vi "Read Theme Data.vi"(8 "error in (no error)":errorcluster, 11 "Appearance Actor in":refnum<class "Appearance Actor.lvclass">) -> (0 "error out":errorcluster, 2 "Theme Data":T1, 3 "Appearance Actor out":refnum<class "Appearance Actor.lvclass">)   [LabVIEW 2021, in "Appearance Actor.lvlib" / "Appearance Actor.lvclass"]
uses:
  Appearance Actor.lvclass
  Typedefs/Theme Data--cluster.ctl
  <vilib>/Utility/config.llb/Config Data RefNum.ctl
  Appearance Actor.lvclass/Appearance Actor.ctl
  <vilib>/Utility/config.llb/NI_LVConfig.lvlib
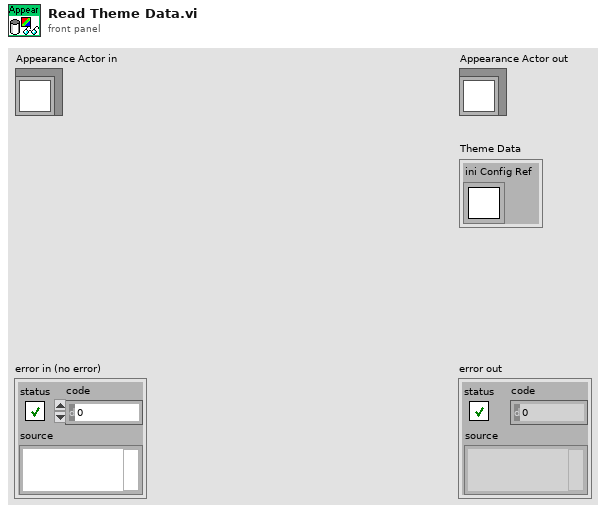
[diagram p1: front panel]
types:
  T1 = typedef "Appearance Actor.lvlib/Appearance Actor.lvclass/Theme Data--cluster.ctl" = cluster{"ini Config Ref":T2}
  T2 = typedef "NI_LVConfig.lvlib/Config Data RefNum.ctl" = refnum<k1>
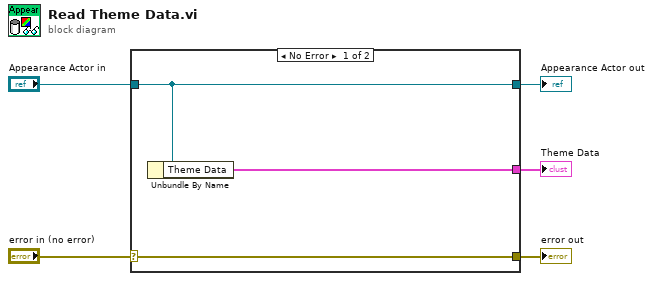
[diagram p0: block diagram]
diagram:
  n1 = case shown="No Error" "error in (no error)" {
    selector: "error in (no error)" -> [w8 w9]
    tunnel: [w8 w9] -> w4
    tunnel: [w7 w10] -> w2
    tunnel: "Appearance Actor in" -> [w7 w10]
    tunnel: [w6 _] -> w1
    frame No Error {
      n2 = Unbundle By Name(w7) -> ("Theme Data"=w6:T1)
    }
    frame Error {
    }
  }
  "error out" <- w4
  "Appearance Actor out" <- w2
  "Theme Data" <- w1
